vi "F-70 controller main.vi"() -> ()   [LabVIEW 2021, in "Magnet module.lvlib" / "F-70 controller.lvlib"]
uses:
  F-70 controller.lvlib
  controls/F-70 controller states.ctl
panel:
  in  "Start Stop btn":bool
  in  "Connect btn":bool
  in  "VISA resource name":refnum<visa-resource-name>
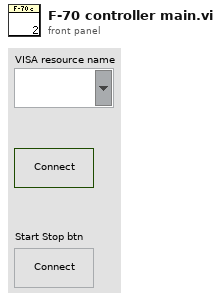
[diagram p1: front panel]
types:
  T1 = typedef "Magnet module.lvlib/F-70 controller.lvlib/F-70 controller states.ctl" = enum16{"Initialize GUI", "Wait for event", "Check message", "Execute command", "Send response", "Sleep", "Reserved", "Reserved2", "End"}
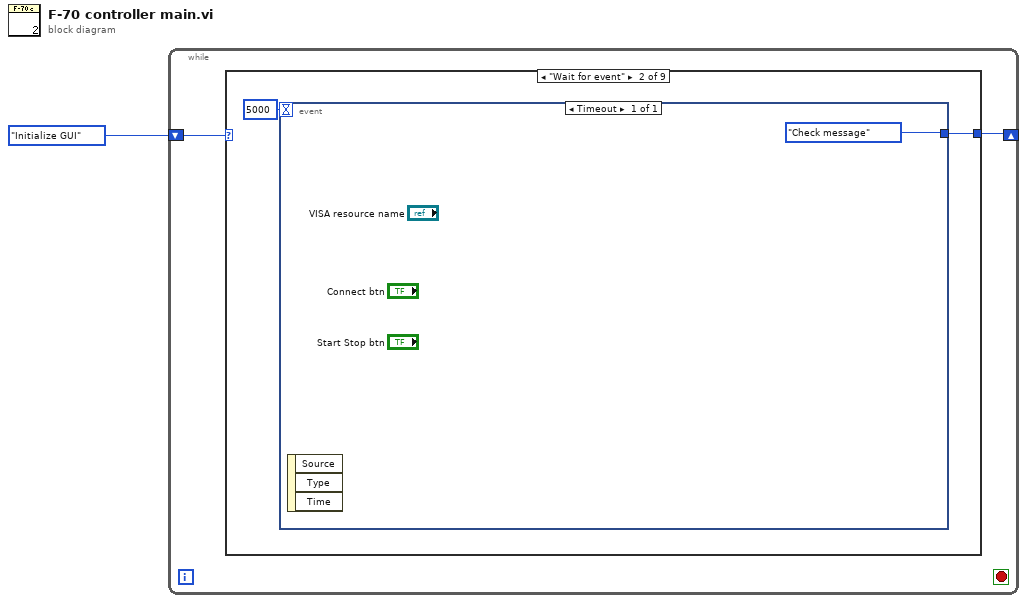
[diagram p0: block diagram]
diagram:
  n1 = while {
    shift-right: [w2] -> _
    shift-left: F-70_controller_states."Initialize GUI" -> [w3]
    stop <- _ stop-if-true
    n2 = case shown="\"Wait for event\"" w3 {
      tunnel: [_ w4 _ _ _ _ _ _ _] -> w2
      frame "Initialize GUI", Default {
      }
      frame "Wait for event" {
        n3 = event shown="[0] Timeout" {
          selector: _ -> [_]
          dyn-events: _ -> [_]
          timeout: 5000 -> [_]
          tunnel: [F-70_controller_states."Check message"] -> w4
          event Timeout {
            n4 = event-data() -> ()  [unwired: 1 in, 3 out]
          }
        }
      }
      frame "Check message" {
      }
      frame "Execute command" {
      }
      frame "Send response" {
      }
      frame "Sleep" {
      }
      frame "Reserved" {
      }
      frame "Reserved2" {
      }
      frame "End" {
      }
    }
  }
